vi "TimerVI.vi"(7 "TimerAction(Read)":enum16{"StartTimer", "ReadTimer"}(ring), 8 "error in (no error)":errorcluster, 11 "TargetTime(mS)":dbl) -> (0 "error out":errorcluster, 1 "TimeLapsed?":bool, 3 "TimeLapsed(mS)":dbl)   [LabVIEW 2023, in "HardwareAbstractionLayer_LVOOP.lvlib" / "CAN Application Protocols Lib.lvlib" / "STP Protocol.lvclass"]
uses:
  STP Protocol.lvclass
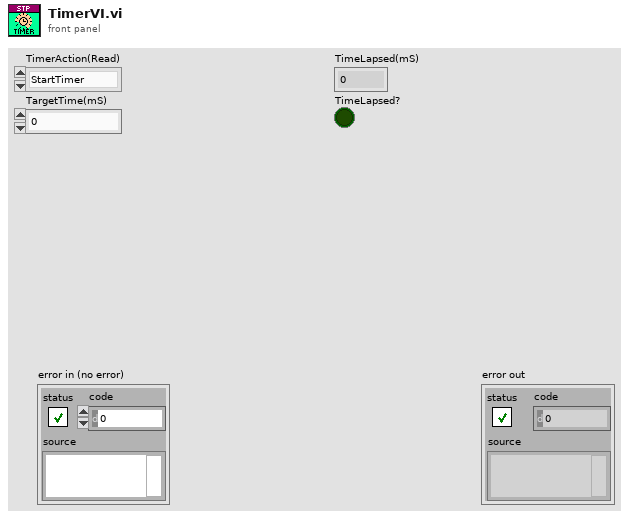
[diagram p1: front panel]
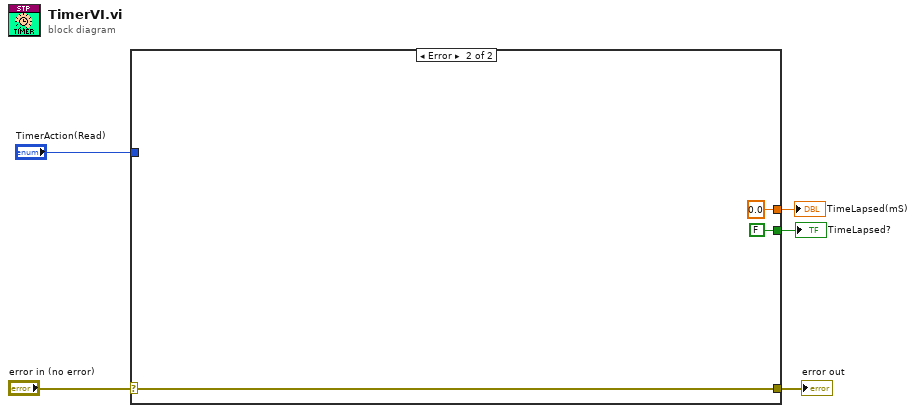
[diagram p0: block diagram]
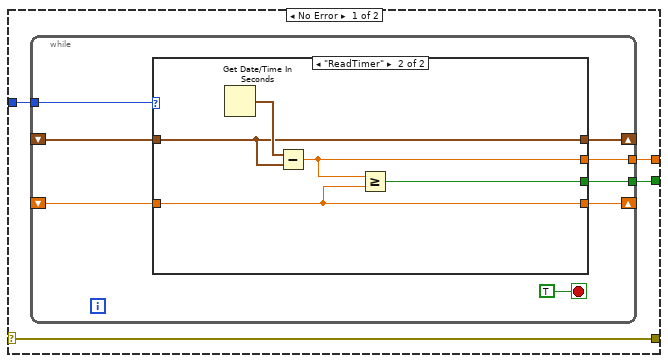
[diagram p2: hidden frame]
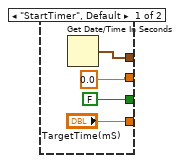
[diagram p3: hidden frame]
diagram:
  n1 = case shown="Error" "error in (no error)" {
    selector: "error in (no error)" -> [w9 w29]
    tunnel: [w9 w29] -> w4
    tunnel: "TimerAction(Read)" -> [w8 _]
    tunnel: [w7 0.0] -> w2
    tunnel: [w6 FALSE] -> w1
    frame No Error {
      n2 = while {
        tunnel: w8 -> [w16]
        shift-right: [w15] -> _
        shift-left: _ -> [w14]
        tunnel: [w13] -> w7
        shift-right: [w12] -> _
        shift-left: _ -> [w11]
        tunnel: [w10] -> w6
        stop <- TRUE stop-if-true
        n3 = case shown="\"ReadTimer\"" w16 {
          tunnel: [w21 w25] -> w15
          tunnel: w14 -> [_ w25]
          tunnel: [0.0 w24] -> w13
          tunnel: ["TargetTime(mS)" w23] -> w12
          tunnel: w11 -> [_ w23]
          tunnel: [FALSE w22] -> w10
          frame "StartTimer", Default {
            n4 = Get Date/Time In Seconds() -> (seconds since 1Jan1904=w21:timestamp)
          }
          frame "ReadTimer" {
            n5 = Get Date/Time In Seconds() -> (seconds since 1Jan1904=w26:timestamp)
            n6 = Subtract(x=w26, y=w25) -> (x-y=w24:dbl)
            n7 = Greater Or Equal?(x=w24, y=w23) -> (x >= y?=w22:bool)
          }
        }
      }
    }
    frame Error {
    }
  }
  "error out" <- w4
  "TimeLapsed(mS)" <- w2
  "TimeLapsed?" <- w1
